vi "FileStream Initialize.vi"(8 "error in (no error)":errorcluster, 9 "mode":i32(ring)=1 items=["CreateNew"=1, "Create"=2, "Open"=3, "OpenOrCreate"=4, "Truncate"=5, "Append"=6], 11 "path":path) -> (0 "error out":errorcluster, 3 "new reference":refnum<k24>)   [LabVIEW 2017, in "File Stream.lvlib"]
doc: "Initializes a new instance of the FileStream class with the specified path and creation mode."
uses:
  File Stream.lvlib
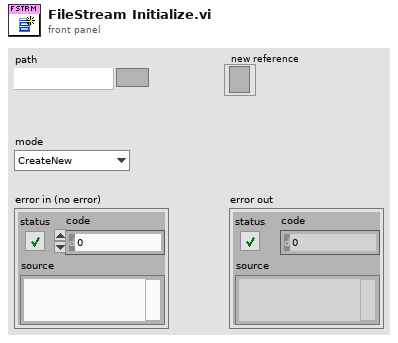
[diagram p1: front panel]
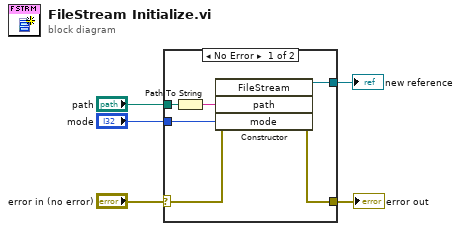
[diagram p0: block diagram]
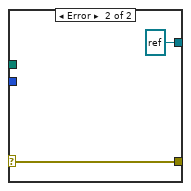
[diagram p2: hidden frame]
diagram:
  n1 = case shown="No Error" "error in (no error)" {
    selector: "error in (no error)" -> [w8 w13]
    tunnel: "mode" -> [w10 _]
    tunnel: "path" -> [w9 _]
    tunnel: [w7 refnum<k24> refnum ("new reference")] -> w2
    tunnel: [w6 w13] -> w1
    frame No Error {
      n2 = Path To String(path=w9) -> (string=w11:string)
      n3 = constructor class="FileStream"(error in=w8, "path"=w11, "mode"=w10) -> (reference out=w7:refnum<k24>, error out=w6:errorcluster)  [unwired: 2 in, 3 out]
    }
    frame Error {
    }
  }
  "new reference" <- w2
  "error out" <- w1
